vi "GetLimsTestStepsAcquisitions.vi"(8 "error in (no error)":errorcluster, 10 "test-id":i32, 11 "ByteGSAPIBase in":refnum<class "ByteGSAPIBase.lvclass">) -> (0 "error out":errorcluster, 2 "list of steps":T1[](array[typedef]), 3 "ByteGSAPIBase out":refnum<class "ByteGSAPIBase.lvclass">)   [LabVIEW 2019, in "ByteGSWebAPI.lvlib" / "ByteGSAPIBase.lvclass"]
doc: "Obtain the list of steps for a Test based on the test-id"
uses:
  ByteGSAPIBase.lvclass
  TypeDef/Step.ctl
  TypeDef/Asset.ctl
  TypeDef/StepAcquisition.ctl
  ByteGSAPIBase.lvclass/ByteGSAPIBase.ctl
  <vilib>/Bytelabs/ByteREST/ByteRESTClass/ByteRESTBase/RESTBase.lvclass
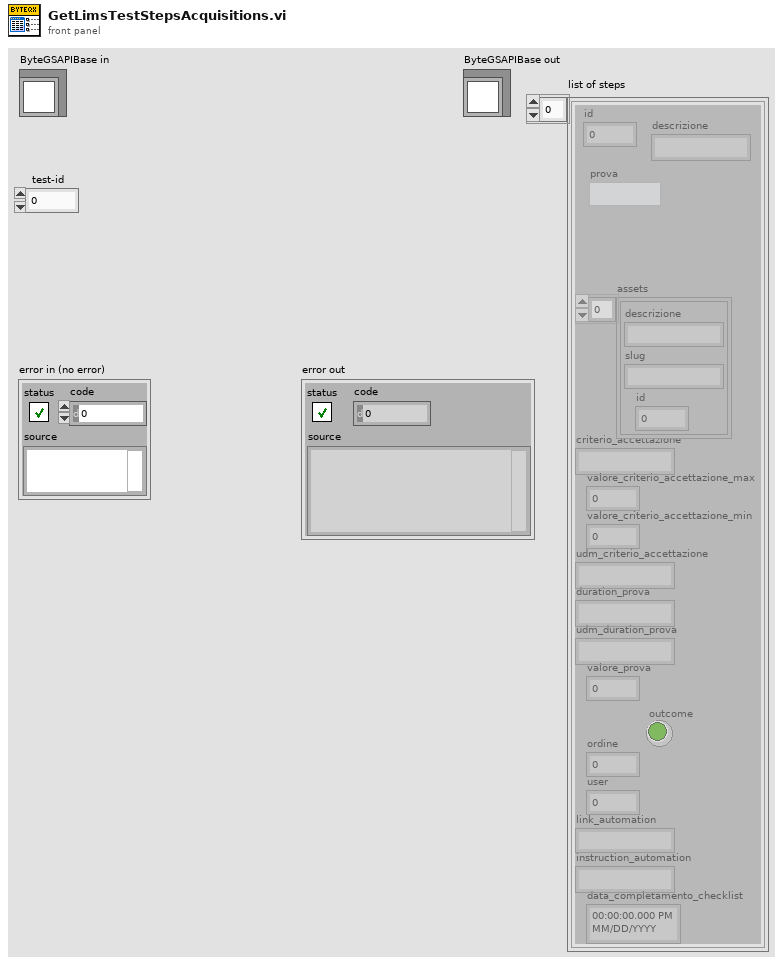
[diagram p1: front panel]
types:
  T1 = typedef "ByteGSWebAPI.lvlib/ByteGSAPIBase.lvclass/Step.ctl" = cluster{"id":i32, "descrizione":string, "prova":string, "assets":T2[], "criterio_accettazione":string, "valore_criterio_accettazione_max":dbl, "valore_criterio_accettazione_min":dbl, "udm_criterio_accettazione":string, "duration_prova":string, "udm_duration_prova":string, "valore_prova":dbl, "ordine":i32, "user":i32, "link_automation":string, "instruction_automation":string, "data_completamento_checklist":timestamp, "outcome":bool}
  T2 = typedef "ByteGSWebAPI.lvlib/ByteGSAPIBase.lvclass/Asset.ctl" = cluster{"descrizione":string, "slug":string, "id":i32}
  T3 = typedef "ByteGSWebAPI.lvlib/ByteGSAPIBase.lvclass/StepAcquisition.ctl" = cluster{"id":i32, "descrizione":string, "prova":cluster{"slug":string}, "assets":T2[], "criterio_accettazione":string, "valore_criterio_accettazione_max":dbl, "valore_criterio_accettazione_min":dbl, "udm_criterio_accettazione":string, "duration_prova":string, "udm_duration_prova":string, "valore_prova":dbl, "ordine":i32, "user":i32, "link_automation":string, "instruction_automation":string, "data_completamento_checklist":timestamp, "outcome":bool, "step_type":string, "channels":string[]}
  T4 = cluster{"id":i32, "descrizione":string, "prova":cluster{"slug":string}, "assets":T2[], "criterio_accettazione":string, "valore_criterio_accettazione_max":dbl, "valore_criterio_accettazione_min":dbl, "udm_criterio_accettazione":string, "duration_prova":string, "udm_duration_prova":string, "data_completamento_checklist":string, "valore_prova":dbl, "outcome":string, "ordine":i32, "user":i32, "link_automation":string, "instruction_automation":string}[]
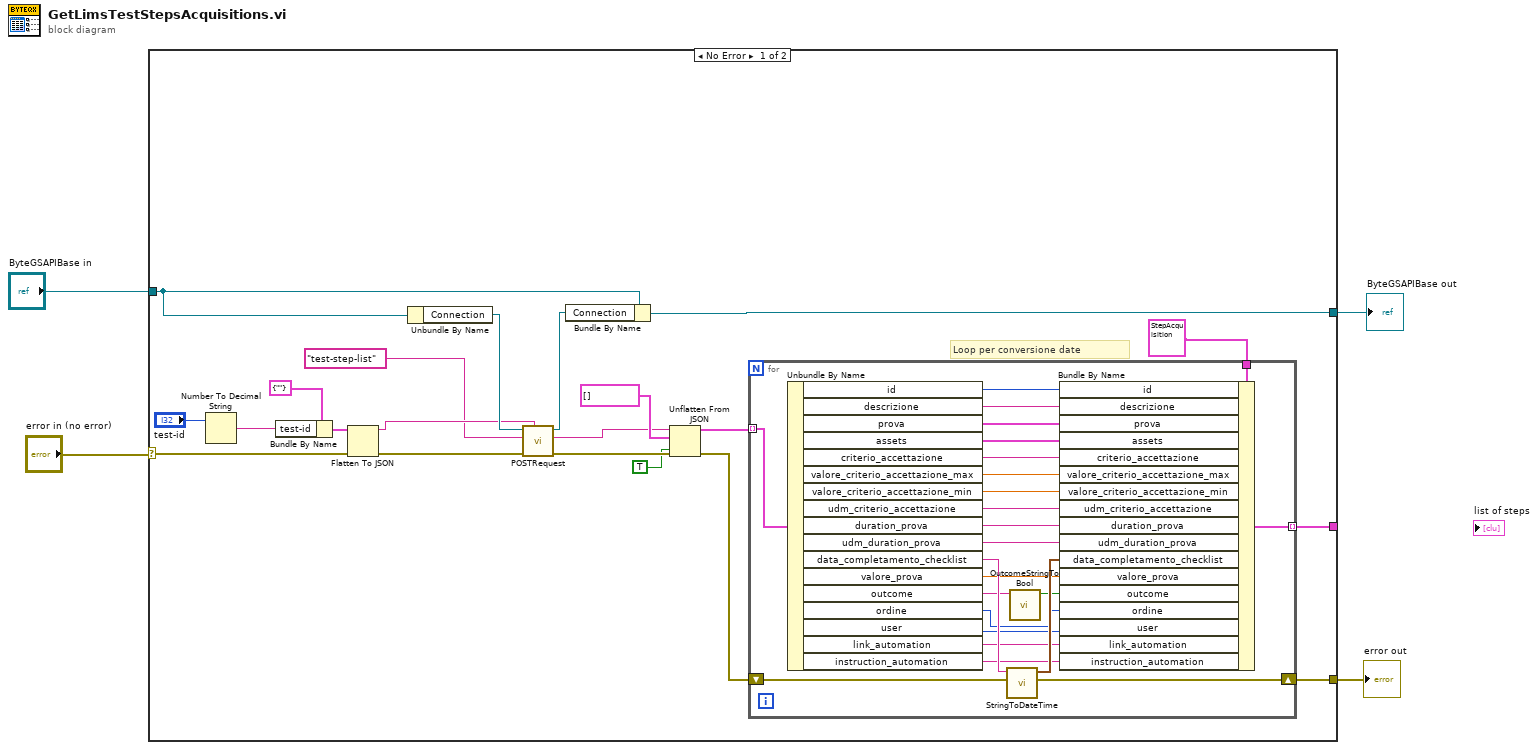
[diagram p0: block diagram]
diagram:
  n1 = case shown="No Error" "error in (no error)" {
    selector: "error in (no error)" -> [w22 w51]
    tunnel: [w8 w51] -> w3
    tunnel: [w23 w50] -> w1
    tunnel: "ByteGSAPIBase in" -> [w14 w50]
    tunnel: [w6 _] -> _
    frame No Error {
      # "Loop per conversione date"
      n2 = Number To Decimal String(number="test-id") -> (decimal integer string=w12:string)  [unwired: 1 in]
      n3 = Bundle By Name(cluster=cluster{"test-id":string} {"test-id"=""} ("Request"), "test-id"=w12) -> (w11:cluster{"test-id":string})
      n4 = Flatten To JSON(anything=w11, error in (no error)=w22) -> (JSON string=w20:string, 11:w24:errorcluster)  [unwired: 1 in]
      n5 = Unbundle By Name(w14) -> ("Connection"=w25:refnum<class "RESTBase.lvclass">)
      n6 = call-dynamic "POSTRequest.vi"("Body in"=w20, "error in (no error)"=w24, "Request"="test-step-list", "ByteRESTBase in"=w25) -> ("error out"=w18:errorcluster, "Body"=w16:string, "ByteRESTBase out"=w17:refnum<class "RESTBase.lvclass">)  [unwired: 4 in, 1 out]
      n7 = Bundle By Name(cluster=w14, "Connection"=w17) -> (w23:refnum<class "ByteGSAPIBase.lvclass">)
      n8 = Unflatten From JSON(JSON string=w16, type and defaults=T4 [], default null elements? (F)=TRUE, error in (no error)=w18) -> (value=w10:T4, error out=w9:errorcluster)  [unwired: 3 in]
      n9 = for {
        tunnel: w10 -> [w49] mode=indexing
        tunnel: T3 {"id"=0, "descrizione"="", "prova"={"slug"=""}, "assets"=[], "criterio_accettazione"="", "valore_criterio_accettazione_max"=0.0, "valore_criterio_accettazione_min"=0.0, "udm_criterio_accettazione"="", "duration_prova"="", "udm_duration_prova"="", "valore_prova"=0.0, "ordine"=0, "user"=0, "link_automation"="", "instruction_automation"="", "data_completamento_checklist"=timestamp(0 s since 1904-01-01), "outcome"=FALSE, "step_type"="", "channels"=[]} ("StepList") -> [w48]
        shift-right: [w29] -> w8
        shift-left: w9 -> [w30]
        tunnel: [w28] -> w6 mode=indexing
        n10 = Unbundle By Name(w49) -> ("id"=w47:i32, "descrizione"=w46:string, "prova"=w45:cluster{"slug":string}, "assets"=w44:T2[], "criterio_accettazione"=w43:string, "valore_criterio_accettazione_max"=w42:dbl, "valore_criterio_accettazione_min"=w41:dbl, "udm_criterio_accettazione"=w40:string, "duration_prova"=w39:string, "udm_duration_prova"=w38:string, "data_completamento_checklist"=w37:string, "valore_prova"=w35:dbl, "outcome"=w27:string, "ordine"=w34:i32, "user"=w33:i32, "link_automation"=w32:string, "instruction_automation"=w31:string)
        n11 = call "StringToDateTime.vi"("error in (no error)"=w30, "datetime string"=w37) -> ("error out"=w29:errorcluster, "timestamp"=w36:timestamp)  [unwired: 8 in]
        n12 = call "OutcomeStringToBool.vi"("outcome string"=w27) -> ("outcome bool"=w26:bool)  [unwired: 10 in]
        n13 = Bundle By Name(cluster=w48, "id"=w47, "descrizione"=w46, "prova"=w45, "assets"=w44, "criterio_accettazione"=w43, "valore_criterio_accettazione_max"=w42, "valore_criterio_accettazione_min"=w41, "udm_criterio_accettazione"=w40, "duration_prova"=w39, "udm_duration_prova"=w38, "data_completamento_checklist"=w36, "valore_prova"=w35, "outcome"=w26, "ordine"=w34, "user"=w33, "link_automation"=w32, "instruction_automation"=w31) -> (w28:T3)
      }
    }
    frame Error {
    }
  }
  "error out" <- w3
  "ByteGSAPIBase out" <- w1
